vi "ini_save_string_vector.vi"(7 "section":string, 8 "error in":errorcluster, 9 "values":string[](array[string]), 10 "key":string, 11 "refnum in":T1) -> (0 "error out":errorcluster, 2 "found?":bool, 3 "refnum out":T1)   [LabVIEW 2020]
uses:
  <vilib>/Utility/config.llb/Config Data RefNum.ctl
  <vilib>/Utility/config.llb/Write Key (String).vi
  <vilib>/Utility/config.llb/NI_LVConfig.lvlib
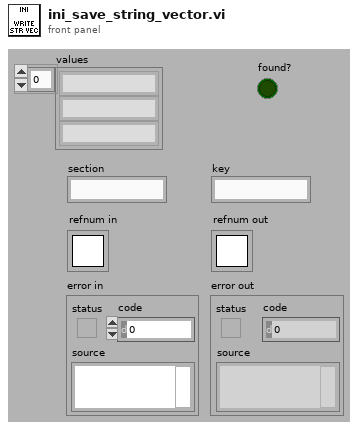
[diagram p1: front panel]
types:
  T1 = typedef "NI_LVConfig.lvlib/Config Data RefNum.ctl" = refnum<k1>
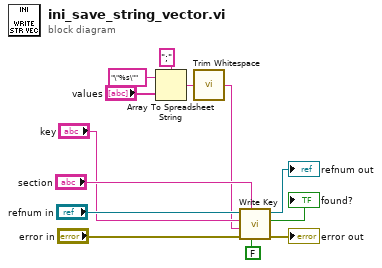
[diagram p0: block diagram]
diagram:
  n1 = Array To Spreadsheet String(delimiter (Tab)=";", array="values", 3:"\"%s\"" ("format string")) -> (spreadsheet string=w5:string)
  n2 = call <vilib>:"Trim Whitespace.vi"("string"=w5) -> ("trimmed string"=w2:string)  [unwired: 1 in]
  n3 = call-poly <vilib>:"Write Key.vi"("write raw string? (F)"=FALSE, "section"="section", "error in (no error)"="error in", "value"=w2, "key"="key", "refnum"="refnum in") -> ("error out"=→"error out":errorcluster, "found?"=→"found?":bool, "refnum out"=→"refnum out":T1)  [unwired: 3 in]
